vi "污染物CP编码.vi"(6 "字符串":string="N", 7 "字段结束":bool=TRUE, 8 "数据类型":string(combo)="-Rtd=", 9 "污染物浓度":string, 10 "污染物编码":string) -> (3 "编码输出":string)   [LabVIEW 2016, in "数据传输系统.lvlib"]
panel:
  # "302-Min=7.220,302-Avg=7.251,302-Max=7.274,302-Flag=N"
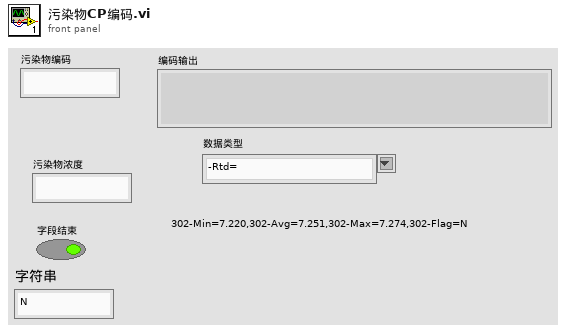
[diagram p1: front panel]
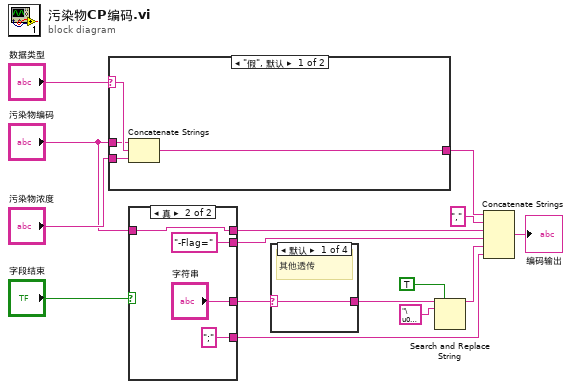
[diagram p0: block diagram]
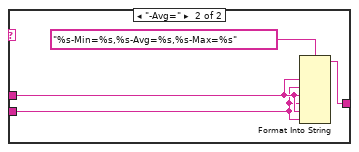
[diagram p2: hidden frame]
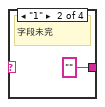
[diagram p3: hidden frame]
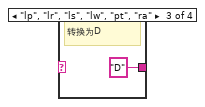
[diagram p4: hidden frame]
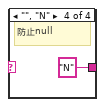
[diagram p5: hidden frame]
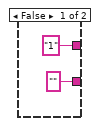
[diagram p6: hidden frame]
diagram:
  n1 = case shown="\"假\", 默认" "数据类型" {
    selector: "数据类型" -> [w19 _]
    tunnel: [w17 w20] -> w3
    tunnel: "污染物浓度" -> [w18 w21]
    tunnel: "污染物编码" -> [w16 w22]
    frame "假", Default {
      n2 = Concatenate Strings(w16, w19, w18) -> (w17:string)
    }
    frame "-Avg=" {
      n3 = Format Into String(format string="%s-Min=%s,%s-Avg=%s,%s-Max=%s" ("格式字符串"), w22, w21, w22, w21, w22, w21) -> (resulting string=w20:string)  [unwired: 2 in, 1 out]
    }
  }
  n4 = case shown="真" "字段结束" {
    tunnel: [_ "-Flag=" ("字符串")] -> w13
    tunnel: ["1" ("字符串") "字符串"] -> w10
    tunnel: "污染物编码" -> [_ w28]
    tunnel: [_ w28] -> w11
    tunnel: ["" ("字符串") ";" ("字符串")] -> w5
    frame False {
    }
    frame True {
    }
  }
  n5 = case shown="默认" w10 {
    selector: w10 -> [w30 _ _ _]
    tunnel: [w30 "" ("字符串") "D" ("字符串") "N" ("字符串")] -> w9
    frame Default {
      # "其他透传"
    }
    frame "1" {
      # "字段未完"
    }
    frame "lp", "lr", "ls", "lw", "pt", "ra" {
      # "转换为D"
    }
    frame "", "N" {
      # "防止null"
    }
  }
  n6 = Search and Replace String(replace all?=TRUE ("替换全部？(F)"), input string=w9, search string="\u0000" ("搜索字符串")) -> (result string=w7:string)  [unwired: 5 in, 3 out]
  n7 = Concatenate Strings(w3, "," ("字符串"), w11, w13, w7, w5) -> (→"编码输出":string)
